vi "Main.vi"() -> ()   [LabVIEW 2015]
doc: "This template is for the Queued Message Handler design pattern.\n\nThe Event Handling Loop generates messages based on user interface actions.\n\nThe Message Handling Loop processes messages generated by the Event Handling Loop, or by other messages. The messages are string values, so new messages can be added easily to the Message Cases case structure in the Message Handling Loop. Each message cluster can also provide an optional value for Message Data, which is a variant that can be converted to whatever message-specific data is required."
uses:
  controls/UI Data.ctl
  support/Message Queue/Enqueue Message (Single).vi
  <vilib>/Utility/error.llb/Error Cluster From Error Code.vi
  <vilib>/ErrorRing/Error Ring.xnode
  support/Message Queue/Message Queue.lvlib
  support/User Event - Stop/User Event - Stop.lvlib
panel:
  out "Progress":u8(slide) scale=0.0..100.0
  in  "End":bool
  in  "Start":bool
  out "Work time 2":string="00:00:00"
  out "Work time":string="00:00:00"
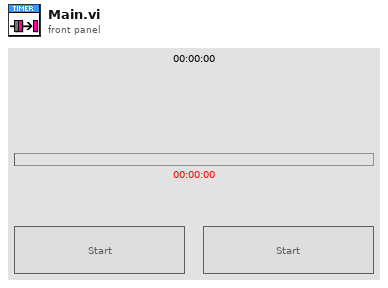
[diagram p1: front panel]
types:
  T1 = typedef "UI Data.ctl" = cluster{"PLACEHOLDER":dbl}
  T2 = typedef "Message Queue.lvlib/All Message Queues.ctl" = cluster{"Main":refnum<queue>, "GUI":refnum<queue>}
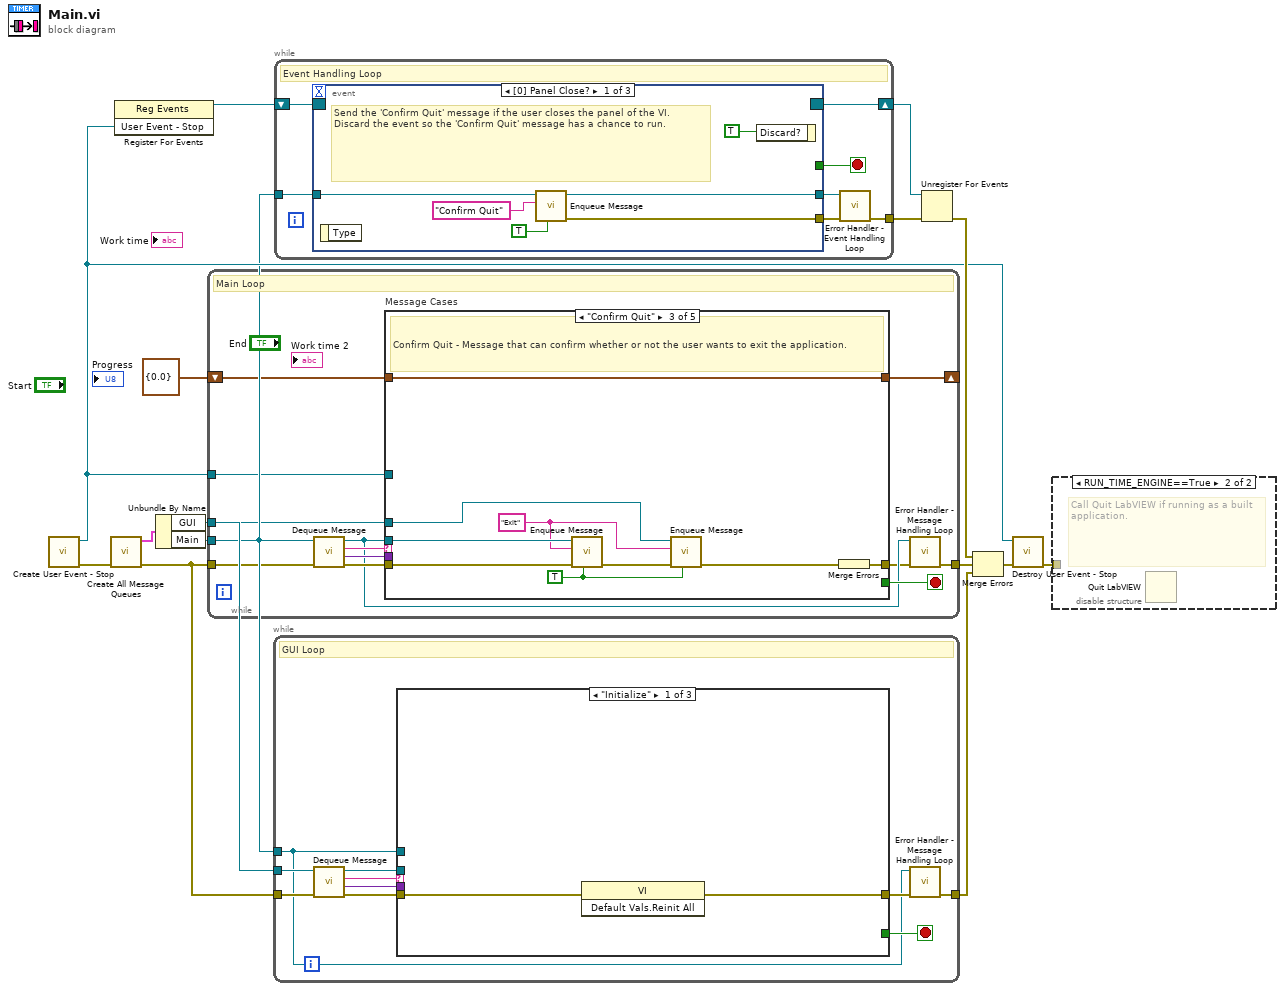
[diagram p0: block diagram]
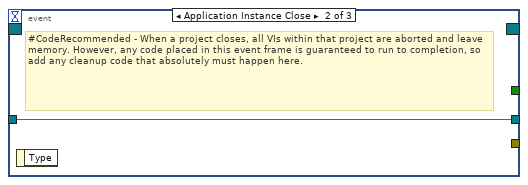
[diagram p3: hidden frame]
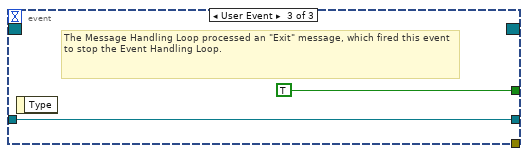
[diagram p4: hidden frame]
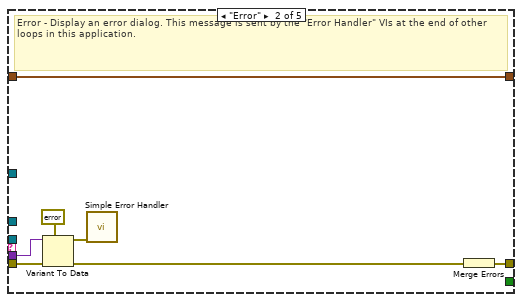
[diagram p6: hidden frame]
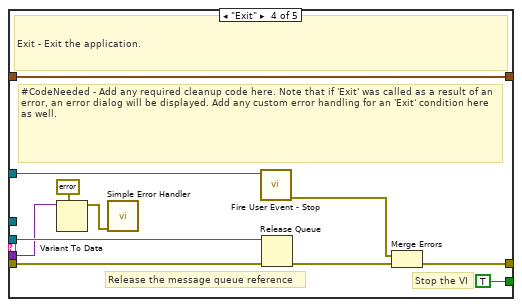
[diagram p7: hidden frame]
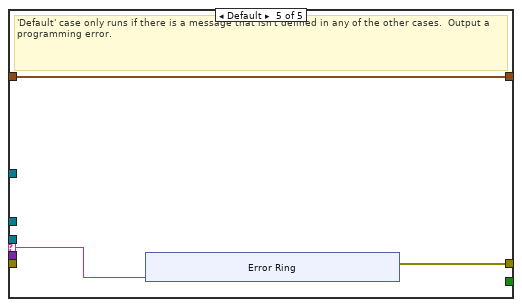
[diagram p8: hidden frame]
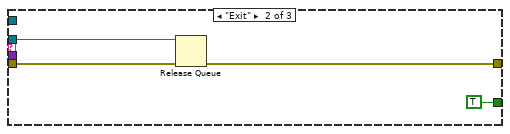
[diagram p9: hidden frame]
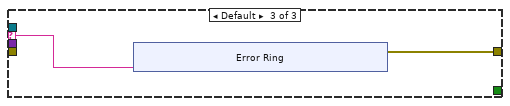
[diagram p10: hidden frame]
diagram:
  n1 = call "Create User Event - Stop.vi"() -> ("error out"=w13:errorcluster, "User Event - Stop"=w5:refnum<user-event>)  [unwired: 10 in]
  n2 = call "Create All Message Queues.vi"("error in (no error)"=w13) -> ("error out"=w4:errorcluster, "Message Queues out"=w15:T2)  [unwired: 9 in]
  n3 = register-events(w5) -> (reference out=w6:refnum<event-registration>)  [unwired: 2 in, 1 out]
  n4 = Unbundle By Name(w15) -> ("GUI"=w3:refnum<queue>, "Main"=w2:refnum<queue>)
  n5 = while {
    tunnel: w2 -> [w20]
    shift-right: [w27] -> _
    shift-left: T1 {"PLACEHOLDER"=0.0} ("Data Cluster") -> [w28]
    tunnel: w5 -> [w25]
    tunnel: w4 -> [w24]
    tunnel: [w18] -> w14
    tunnel: w3 -> [w16]
    stop <- w26 stop-if-true
    # "Main Loop"
    n6 = call "Dequeue Message.vi"("error in (no error)"=w24, "Message Queue"=w20) -> ("error out"=w23:errorcluster, "Message Data"=w21:variant, "Message"=w22:string, "dup Message Queue"=w19:refnum<queue>)  [unwired: 6 in]
    n7 = case "Message Cases" shown="\"Confirm Quit\"" w22 {
      selector: w22 -> [_ _ _ _ w58]
      tunnel: w19 -> [_ _ w43 w57 _]
      tunnel: w23 -> [w30 w37 w46 w50 _]
      tunnel: [w30 w31 w44 w53 w59] -> w17
      tunnel: w28 -> [w29 w36 w45 w56 w60]
      tunnel: [w29 w36 w45 w56 w60] -> w27
      tunnel: [_ _ _ TRUE _] -> w26
      tunnel: w21 -> [_ w35 _ w47 _]
      tunnel: w25 -> [_ _ _ w52 _]
      tunnel: w16 -> [_ _ w39 _ _]
      frame "Initialize" {
        # "Initialize - All initialization work should take place in this message, since other loops can potentially enqueue messages that execute immediately after this one."
      }
      frame "Error" {
        # "Error - Display an error dialog. This message is sent by the \"Error Handler\" VIs at the end of other loops in this application."
        n8 = Variant To Data(error in=w37, type=errorcluster {"status"=FALSE, "code"=0, "source"=""} ("error constant"), Variant=w35) -> (data=w33:errorcluster, error out=w32:errorcluster)
        n9 = call <vilib>:"Simple Error Handler.vi"("error in (no error)"=w33) -> ()  [unwired: 4 in, 5 out]
        n10 = Merge Errors(w32) -> (w31:errorcluster)
      }
      frame "Confirm Quit" {
        w40 = "Exit" ("Message")
        w41 = TRUE ("Priority Message? (F)")
        # "Confirm Quit - Message that can confirm whether or not the user wants to exit the application."
        n11 = call-poly "Enqueue Message.vi"("Priority Message? (F)"=w41, "error in (no error)"=w46, "Message"=w40, "Message Queue"=w43) -> ("error out"=w42:errorcluster)  [unwired: 6 in, 1 out]
        n12 = call-poly "Enqueue Message.vi"("Priority Message? (F)"=w41, "error in (no error)"=w42, "Message"=w40, "Message Queue"=w39) -> ("error out"=w38:errorcluster)  [unwired: 6 in, 1 out]
        n13 = Merge Errors(w38) -> (w44:errorcluster)
      }
      frame "Exit" {
        # "Stop the VI"
        # "Release the message queue reference"
        # "#CodeNeeded - Add any required cleanup code here. Note that if 'Exit' was called as a result of an error, an error dialog will be displayed. Add any custom error handling for an 'Exit' condition here as well."
        # "Exit - Exit the application."
        n14 = Variant To Data(type=errorcluster {"status"=FALSE, "code"=0, "source"=""} ("error constant"), Variant=w47) -> (data=w48:errorcluster)  [unwired: 1 in, 1 out]
        n15 = call <vilib>:"Simple Error Handler.vi"("error in (no error)"=w48) -> ()  [unwired: 4 in, 5 out]
        n16 = call "Fire User Event - Stop.vi"("User Event - Stop"=w52) -> ("error out"=w51:errorcluster)  [unwired: 10 in]
        n17 = Release Queue(queue=w57, error in (no error)=w50) -> (error out=w54:errorcluster)  [unwired: 1 in, 2 out]
        n18 = Merge Errors(w51, w54) -> (w53:errorcluster)
      }
      frame Default {
        # "'Default' case only runs if there is a message that isn't defined in any of the other cases.  Output a programming error."
        n19 = xnode "Error Ring"("parameter 0"=w58) -> ("error out"=w59:errorcluster)
      }
    }
    n20 = call "Error Handler - Message Handling Loop.vi"("error in (no error)"=w17, "Message Queue"=w19) -> ("dup error in"=w18:errorcluster)  [unwired: 8 in, 1 out]
  }
  n21 = while {
    tunnel: w4 -> [w77]
    tunnel: w3 -> [w76]
    tunnel: [w69] -> w1
    tunnel: w2 -> [w68]
    stop <- w70 stop-if-true
    # "GUI Loop"
    n22 = call "Dequeue Message.vi"("error in (no error)"=w77, "Message Queue"=w76) -> ("error out"=w72:errorcluster, "Message Data"=w74:variant, "Message"=w75:string, "dup Message Queue"=w73:refnum<queue>)  [unwired: 6 in]
    n23 = case shown="\"Initialize\"" w75 {
      selector: w75 -> [_ _ w84]
      tunnel: w74 -> [_ _ _]
      tunnel: w73 -> [_ w81 _]
      tunnel: w72 -> [w79 w82 _]
      tunnel: [w78 w80 w85] -> w71
      tunnel: [_ TRUE _] -> w70
      tunnel: w68 -> [_ _ _]
      frame "Initialize" {
        n24 = invoke class="VI" method="Default Vals.Reinit All"(error in=w79) -> (error out=w78:errorcluster)  [unwired: 2 in, 2 out]
      }
      frame "Exit" {
        n25 = Release Queue(queue=w81, error in (no error)=w82) -> (error out=w80:errorcluster)  [unwired: 1 in, 2 out]
      }
      frame Default {
        n26 = xnode "Error Ring"("parameter 0"=w84) -> ("error out"=w85:errorcluster)
      }
    }
    n27 = call "Error Handler - Message Handling Loop.vi"("error in (no error)"=w71, "Message Queue"=w68) -> ("dup error in"=w69:errorcluster)  [unwired: 8 in, 1 out]
  }
  n28 = while {
    tunnel: w2 -> [w99]
    shift-right: [w97] -> w10
    shift-left: w6 -> [w98]
    tunnel: [w93] -> w7
    stop <- w95 stop-if-true
    # "Event Handling Loop"
    n29 = event shown="[0] Panel Close?" {
      selector: w98 -> [_ _ _]
      dyn-events: [_ _ _] -> w97
      timeout: _ -> [_ _ _]
      tunnel: [_ _ TRUE ("Discard?")] -> w95
      tunnel: w99 -> [w104 w106 w108]
      tunnel: [w103 _ _] -> w96
      tunnel: [w102 w106 w108] -> w94
      event Panel Close? {
        # "Send the 'Confirm Quit' message if the user closes the panel of the VI. Discard the event so the 'Confirm Quit' message has a chance to run."
        n30 = event-data() -> ()  [unwired: 1 in, 1 out]
        n31 = call-poly "Enqueue Message.vi"("Priority Message? (F)"=TRUE, "Message"="Confirm Quit", "Message Queue"=w104) -> ("error out"=w103:errorcluster, "dup Message Queue"=w102:refnum<queue>)  [unwired: 7 in]
        n32 = event-data("Discard?"=TRUE) -> ()  [unwired: 1 in, 1 out]
      }
      event Application Instance Close {
        # "#CodeRecommended - When a project closes, all VIs within that project are aborted and leave memory. However, any code placed in this event frame is guaranteed to run to completion, so add any cleanup code that absolutely must happen here."
        n33 = event-data() -> ()  [unwired: 1 in, 1 out]
      }
      event User Event {
        # "The Message Handling Loop processed an \"Exit\" message, which fired this event to stop the Event Handling Loop."
        n34 = event-data() -> ()  [unwired: 1 in, 1 out]
      }
    }
    n35 = call "Error Handler - Event Handling Loop.vi"("error in (no error)"=w96, "Message Queue"=w94) -> ("dup error in"=w93:errorcluster)  [unwired: 8 in, 1 out]
  }
  n36 = Unregister For Events(event registration refnum=w10, error in=w7) -> (error out=w11:errorcluster)
  n37 = Merge Errors(w11, w14, w1) -> (w12:errorcluster)
  n38 = call "Destroy User Event - Stop.vi"("error in (no error)"=w12, "User Event - Stop"=w5) -> ("error out"=w8:errorcluster)  [unwired: 9 in]
  n39 = disable-structure shown="RUN_TIME_ENGINE==True" {
    disable-tunnel: w8 -> [_ _]
    frame condition #0 (active) {
    }
    frame condition #1 {
      # "Call Quit LabVIEW if running as a built application."
      n40 = Quit LabVIEW() -> ()  [unwired: 1 in]
    }
  }
